vi "CPP_Aeroprobe_TimeSeries-MultiProbe.vi"() -> (5 "Plug in titles":string[](array[string]), 7 "Plug in values":string[](array[string]))   [LabVIEW 2013]
uses:
  Globals/Meas_global.vi
panel:
  in  "Graphs":bool=TRUE
  in  "Downsampler":i32=10
  out "Average Reduction (ms)":dbl
  out "Reduction (ms)":u32
  in  "Calibration Folder Path":path=path "G:/5HoleProbe"
  in  "Correction File Path":path=path "M:/Preferences/Rig_Setups/All_Rigs/TubingCompensation/5HPTubingCorrection12066.xls"
  in  "Apply Phase Correction?":bool=TRUE
  out "DataArray":dbl[](array[numeric])
  out "Zeroes":dbl[](array[numeric])
  in  "Old5HoleProbe?":bool
  # "!! 5-hole 1-5 must be connected to Channels 1-5 !!"
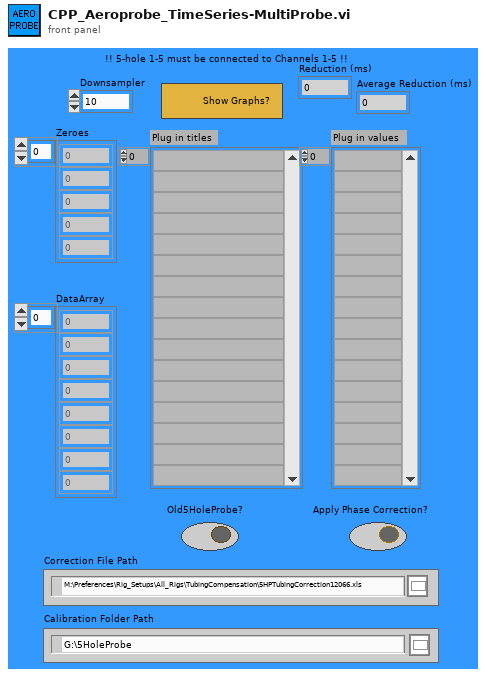
[diagram p1: front panel]
types:
  T1 = typedef "Analysis_info_cluster.ctl" = cluster{"Colour":u32, "Inst type":T2, "Inst name":string, "Symbol":string, "Code name":string, "Extra Info":string, "Inst Array":T3, "Extra Titles":string[], "Extra Values":string[], "U":dbl, "u^2":dbl, "u^3":dbl, "u^4":dbl, "Skew_u":dbl, "Kurt_u":dbl, "Sd Error in Mean":dbl, "% u'/U":dbl, "X":dbl, "Y":dbl, "Z":dbl, "Timescale integral to 25%":dbl, "Sd Error in Variance":dbl, "Calib File":path, "Calib Constants":dbl[], "Output Position":bool, "Full Stats":bool, "Av Sampling Rate":dbl, "Av No of Samples":dbl, "Total Meas Time (s)":dbl, "ADAM Ch Name":string}
  T2 = typedef "Inst_type.ctl" = enum16{"Propeller anemometer", "Raw voltage", "Pressure Transducer", "Pitot-static tube", "Preston tube", "Hot wire", "Cross wire 1", "Cross wire 2", "Generic Linear", "Generic Polynomial", "Generic BackPoly", "Fast FID", "Thermocouple", "Cold wire", "Pulsed Wire", "LDA Vel", "LDA Tran time", "LDA Arr time"}
  T3 = typedef "Instrument_Array.ctl" = enum16{"PWA", "LDA", "Analogue"}
  T4 = cluster{"Analysis Info cluster[0]":T1, "Analysis Info cluster[1]":T1, "Analysis Info cluster[2]":T1, "Analysis Info cluster[3]":T1, "Analysis Info cluster[4]":T1, "Analysis Info cluster[5]":T1, "Analysis Info cluster[6]":T1}
  T5 = typedef "Time_Trace_Cluster.ctl" = cluster{"Weighting":dbl[], "Time (s)":dbl[], "Voltage":dbl[], "Eng Values":dbl[]}
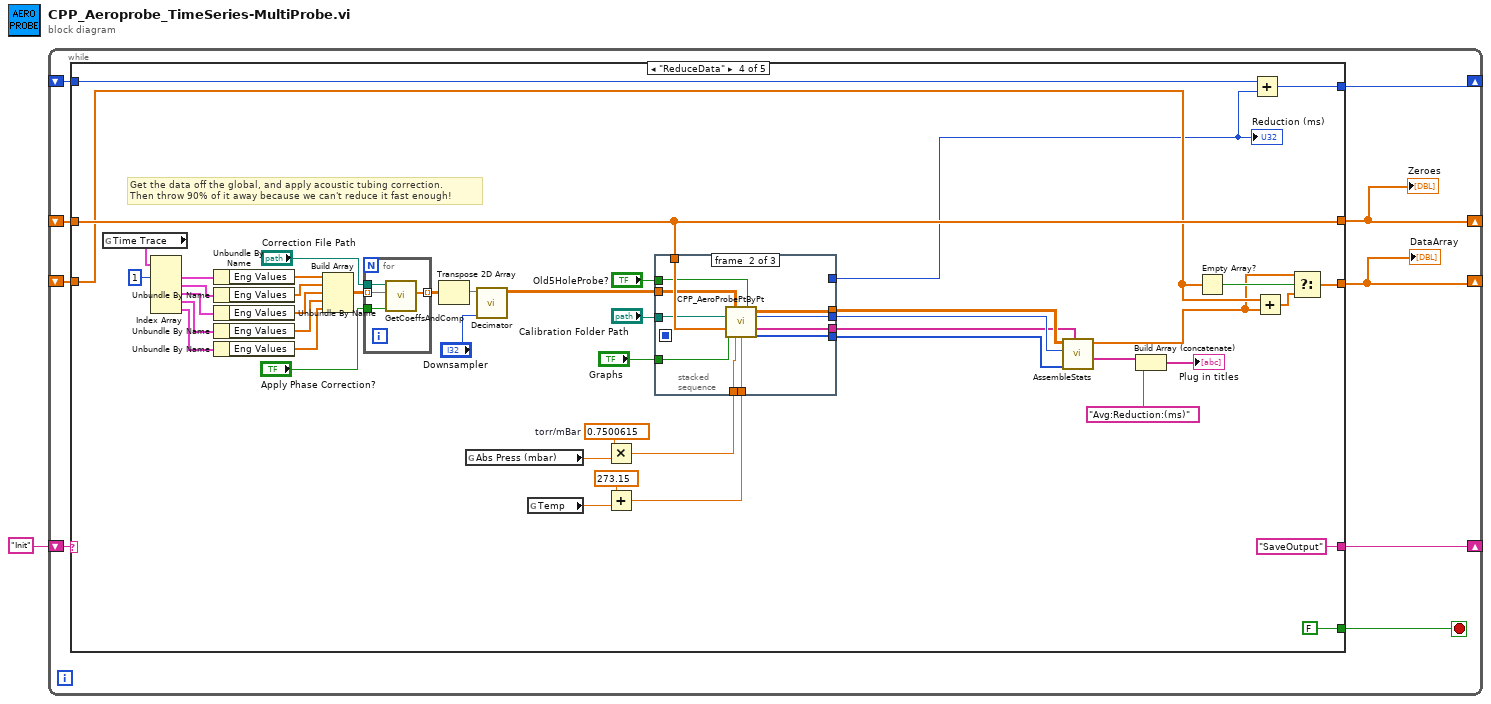
[diagram p0: block diagram]
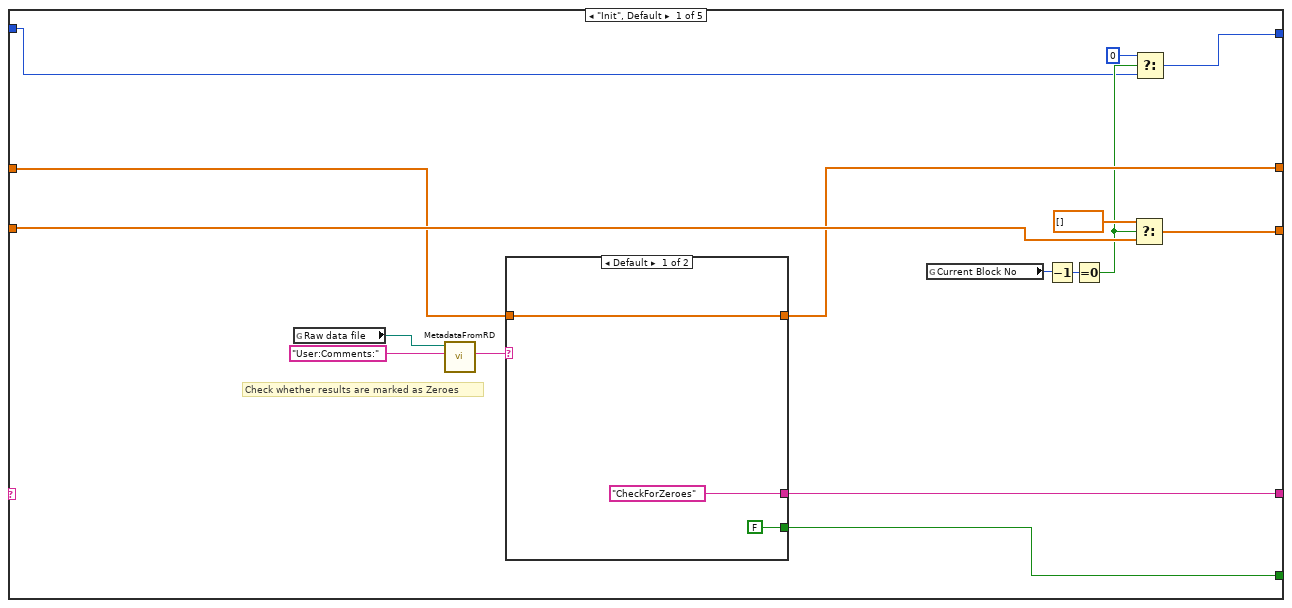
[diagram p2: hidden frame]
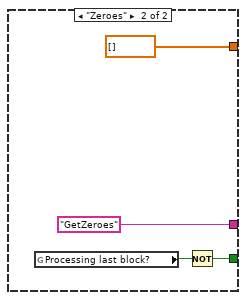
[diagram p3: hidden frame]
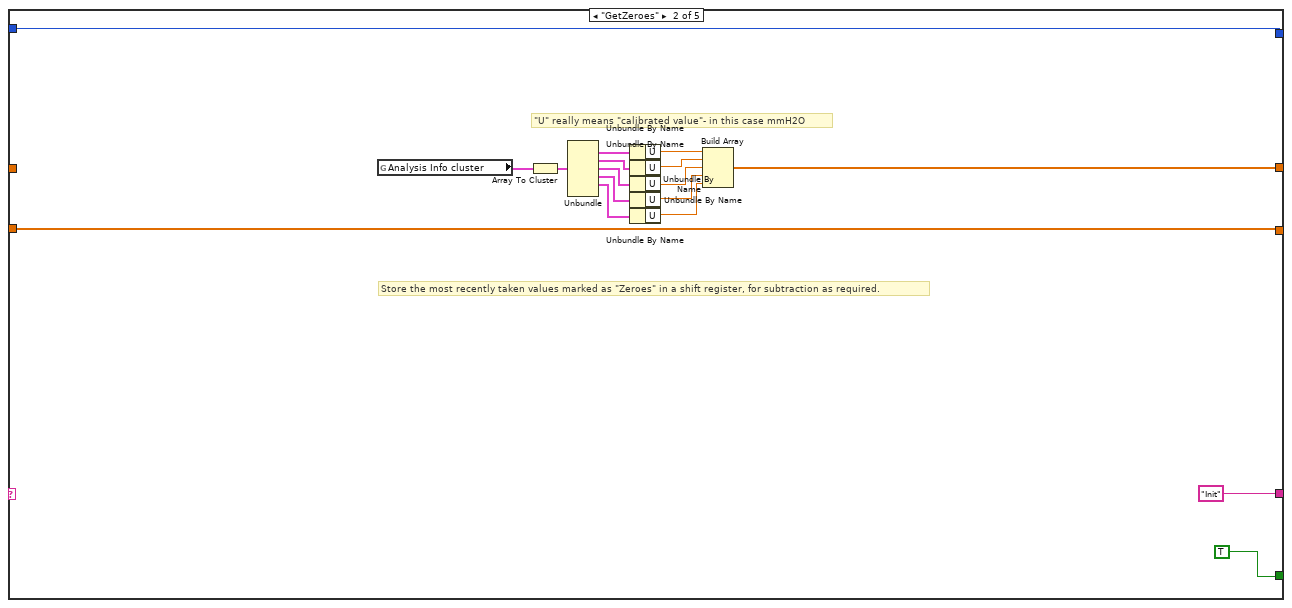
[diagram p4: hidden frame]
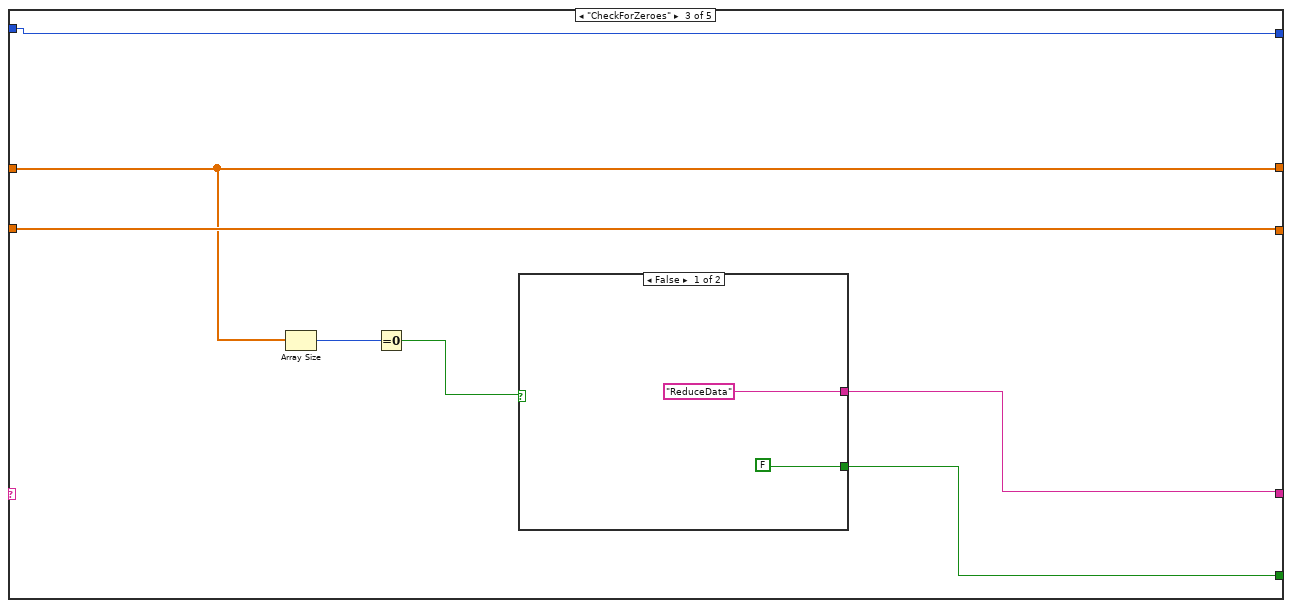
[diagram p5: hidden frame]
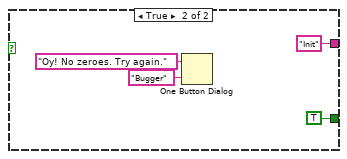
[diagram p6: hidden frame]
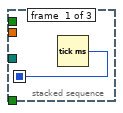
[diagram p7: hidden frame]
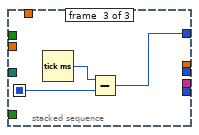
[diagram p8: hidden frame]
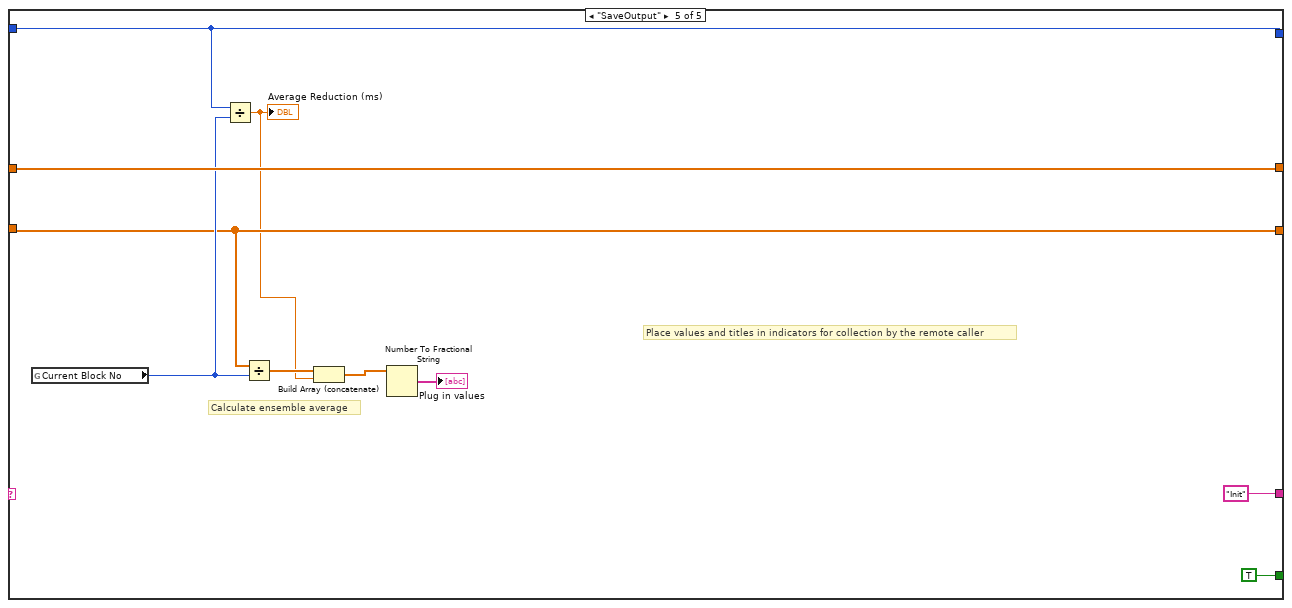
[diagram p9: hidden frame]
diagram:
  n1 = while {
    shift-right: [w9] -> _
    shift-left: "Init" -> [w10]
    shift-right: [w8] -> _
    shift-left: _ -> [w7]
    shift-right: [w6] -> _
    shift-left: _ -> [w5]
    shift-right: [w3] -> _
    shift-left: _ -> [w2]
    stop <- w4 stop-if-true
    n2 = case shown="\"ReduceData\"" w10 {
      tunnel: [w26 "Init" w52 "SaveOutput" "Init"] -> w9
      tunnel: [w17 w37 w55 w108 w138] -> w8
      tunnel: w7 -> [w18 _ w55 w108 w138]
      tunnel: [w20 w35 w56 w91 w131] -> w6
      tunnel: w5 -> [w21 w35 w56 w94 w131]
      tunnel: [w22 TRUE w51 FALSE TRUE] -> w4
      tunnel: [w14 w34 w57 w74 w132] -> w3
      tunnel: w2 -> [w12 w34 w57 w73 w132]
      frame "Init", Default {
        # "Check whether results are marked as Zeroes"
        n3 = global read "Meas_global.vi" "Raw data file"() -> (w25:path)
        n4 = call "MetadataFromRD.vi"("ChannelName"="User:Comments:", "Raw data file"=w25) -> ("ValueString"=w23:string)  [unwired: 8 in, 1 out]
        n5 = case shown="Default" w23 {
          tunnel: ["CheckForZeroes" "GetZeroes"] -> w26
          tunnel: [FALSE w32] -> w22
          tunnel: w18 -> [w27 _]
          tunnel: [w27 dbl[] [] ("t")] -> w17
          frame Default {
          }
          frame "Zeroes" {
            n6 = global read "Meas_global.vi" "Processing last block?"() -> (w31:bool)
            n7 = Not(x=w31) -> (.not. x?=w32:bool)
          }
        }
        n8 = global read "Meas_global.vi" "Current Block No"() -> (w16:i32)
        n9 = Decrement(x=w16) -> (x-1=w15:i32)
        n10 = Equal To 0?(x=w15) -> (x = 0?=w13:bool)
        n11 = Select(t=dbl[] [], s=w13, f=w21) -> (s? t:f=w20:dbl[])
        n12 = Select(t=u32 0, s=w13, f=w12) -> (s? t:f=w14:u32)
      }
      frame "GetZeroes" {
        # "Store the most recently taken values marked as \"Zeroes\" in a shift register, for subtraction as required."
        # "\"U\" really means \"calibrated value\"- in this case mmH2O"
        n13 = global read "Meas_global.vi" "Analysis Info cluster"() -> (w39:T1[])
        n14 = Array To Cluster(array=w39) -> (cluster=w45:T4)
        n15 = Unbundle(w45) -> ("Analysis Info cluster[1]"=w46:T1, "Analysis Info cluster[2]"=w47:T1, "Analysis Info cluster[3]"=w48:T1, "Analysis Info cluster[4]"=w49:T1, "Analysis Info cluster[5]"=w50:T1)  [unwired: 2 out]
        n16 = Unbundle By Name(w46) -> ("U"=w44:dbl)
        n17 = Unbundle By Name(w47) -> ("U"=w43:dbl)
        n18 = Unbundle By Name(w48) -> ("U"=w42:dbl)
        n19 = Unbundle By Name(w49) -> ("U"=w41:dbl)
        n20 = Unbundle By Name(w50) -> ("U"=w40:dbl)
        n21 = Build Array(w44, w43, w42, w41, w40) -> (w37:dbl[])
      }
      frame "CheckForZeroes" {
        n22 = Array Size(array=w55) -> (size(s)=w54:i32)
        n23 = Equal To 0?(x=w54) -> (x = 0?=w53:bool)
        n24 = case shown="False" w53 {
          tunnel: ["ReduceData" "Init"] -> w52
          tunnel: [FALSE TRUE] -> w51
          frame False {
          }
          frame True {
            n25 = One Button Dialog(message="Oy! No zeroes. Try again.", button name ("OK")="Bugger") -> ()  [unwired: 1 out]
          }
        }
      }
      frame "ReduceData" {
        w76 = 0.7500615  # torr/mBar
        # "Get the data off the global, and apply acoustic tubing correction. \nThen throw 90% of it away because we can't reduce it fast enough!"
        n26 = global read "Meas_global.vi" "Time Trace"() -> (w98:T5[])
        n27 = Index Array(array=w98, index #1=1 ("index")) -> (element #1=w97:T5, element #2=w106:T5, element #3=w105:T5, element #4=w104:T5, element #5=w103:T5)  [unwired: 4 in]
        n28 = Unbundle By Name(w97) -> ("Eng Values"=w96:dbl[])
        n29 = Unbundle By Name(w106) -> ("Eng Values"=w102:dbl[])
        n30 = Unbundle By Name(w105) -> ("Eng Values"=w101:dbl[])
        n31 = Unbundle By Name(w104) -> ("Eng Values"=w100:dbl[])
        n32 = Unbundle By Name(w103) -> ("Eng Values"=w99:dbl[])
        n33 = Build Array(w96, w102, w101, w100, w99) -> (w89:dbl[][])
        n34 = for {
          tunnel: w89 -> [w128] mode=indexing
          tunnel: [w127] -> w86 mode=indexing
          tunnel: "Apply Phase Correction?" -> [w126]
          tunnel: "Correction File Path" -> [w125]
          n35 = call "GetCoeffsAndComp.vi"("Apply Phase Correction?"=w126, "mutedData"=w128, "TubingCorrectionFile (pre-set!)"=w125) -> ("boostedData"=w127:dbl[])  [unwired: 8 in]
        }
        n36 = Transpose 2D Array(2D array=w86) -> (transposed array=w85:dbl[][])
        n37 = global read "Meas_global.vi" "Abs Press (mbar)"() -> (w77:dbl)
        n38 = call "Decimator.vi"("Decimator"="Downsampler", "Array In"=w85) -> ("DecimatedArrayOut"=w83:dbl[][])  [unwired: 9 in]
        n39 = global read "Meas_global.vi" "Temp"() -> (w80:dbl)
        n40 = Multiply(x=w76, y=w77) -> (x*y=w75:dbl)
        n41 = Add(x=273.15, y=w80) -> (x+y=w78:dbl)
        n42 = stacked-sequence {
          seq-local: [w110 _ _] -> [_ _ w122]
          tunnel: w83 -> [_ w113 _]
          tunnel: "Graphs" -> [_ w112 _]
          tunnel: w108 -> [_ w121 _]
          tunnel: "Calibration Folder Path" -> [_ w120 _]
          tunnel: "Old5HoleProbe?" -> [_ w119 _]
          tunnel: w78 -> [_ w118 _]
          tunnel: w75 -> [_ w117 _]
          tunnel: [_ w116 _] -> w71
          tunnel: [_ w115 _] -> w68
          tunnel: [_ w114 _] -> w67
          tunnel: [_ _ w124] -> w65
          tunnel: [_ w111 _] -> w64
          frame #0 {
            n43 = Tick Count (ms)() -> (millisecond timer value=w110:u32)
          }
          frame #1 {
            n44 = call "CPP_AeroProbePtByPt.vi"("Data"=w113, "Old5HoleProbe?"=w119, "Calibration Folder Path"=w120, "Zeroes"=w121, "Graphs"=w112, "Pressure (torr)"=w117, "Temperature (K)"=w118) -> ("VmagUVWCone"=w116:dbl[][], "TotalPoints"=w115:i32, "Plug in titles"=w111:string[], "errors"=w114:i16[])  [unwired: 5 in]
          }
          frame #2 {
            n45 = Tick Count (ms)() -> (millisecond timer value=w123:u32)
            n46 = Subtract(x=w123, y=w122) -> (x-y=w124:u32)
          }
        }
        "Reduction (ms)" <- w65
        n47 = call "AssembleStats.vi"("ErrorTitles"=w64, "errors"=w67, "TotalPoints"=w68, "VmagUVWCone"=w71) -> ("Plug in titles"=w72:string[], "StatsArray"=w90:dbl[])  [unwired: 6 in]
        n48 = Build Array (concatenate)(w72, "Avg:Reduction:(ms)") -> (→"Plug in titles":string[])
        n49 = Empty Array?(array=w94) -> (empty?=w93:bool)
        n50 = Add(x=w73, y=w65) -> (x+y=w74:u32)
        n51 = Add(x=w94, y=w90) -> (x+y=w92:dbl[])
        n52 = Select(t=w90, s=w93, f=w92) -> (s? t:f=w91:dbl[])
      }
      frame "SaveOutput" {
        # "Place values and titles in indicators for collection by the remote caller"
        # "Calculate ensemble average"
        n53 = global read "Meas_global.vi" "Current Block No"() -> (w133:i32)
        n54 = Divide(x=w132, y=w133) -> (x/y=w129:dbl)
        "Average Reduction (ms)" <- w129
        n55 = Divide(x=w131, y=w133) -> (x/y=w134:dbl[])
        n56 = Build Array (concatenate)(w134, w129) -> (w130:dbl[])
        n57 = Number To Fractional String(number=w130) -> (F-format string=→"Plug in values":string[])  [unwired: 3 in]
      }
    }
    "Zeroes" <- w8
    "DataArray" <- w6
  }
